vi "Periodic Tasks.vi"(8 "error in":errorcluster) -> ()   [LabVIEW 2018]
doc: "This VI runs in parallel to other tasks. It can contain as many user-defined periodic loops as you need. These can carry out PID or other sorts of timed response."
uses:
  SwerveRotationCalibrate.ctl
  <vilib>/Rock Robotics/WPI/ThirdParty/Phoenix-LabVIEW/Motor Controller/Controls/CTRE_Phoenix_MotorControl_NeutralMode.ctl
  <vilib>/Rock Robotics/WPI/ThirdParty/Phoenix-LabVIEW/Motor Controller/Controls/CTRE_Phoenix_MotorControl_ControlMode.ctl
  <vilib>/Rock Robotics/WPI/ThirdParty/Phoenix-LabVIEW/Motor Controller/Controls/CTRE_Phoenix_MotorControl_FeedbackDevice.ctl
  <vilib>/Rock Robotics/WPI/Utilities/WPI_GetSetVariantRefNum.vi
  <vilib>/Rock Robotics/Network Tables/NT Read Boolean.vi
  Robot Global Data.vi
  <vilib>/Rock Robotics/Network Tables/NT Write Numeric Array.vi
  d8969dce-e83f-414b-ab1b-b6caec8a5545.vi
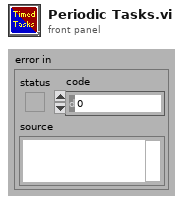
[diagram p1: front panel]
types:
  T1 = typedef "SwerveRotationCalibrate.ctl" = enum16{"Calibrate", "Home", "ResetQuad", "Drive"}
  T2 = typedef "CTRE_Phoenix_MotorControl_NeutralMode.ctl" = enum8{"EEPROMSetting", "Override to Coast", "Override to Brake"}
  T3 = typedef "CTRE_Phoenix_MotorControl_ControlMode.ctl" = u16
  T4 = typedef "CTRE_Phoenix_MotorControl_FeedbackDevice.ctl" = i8
  T5 = cluster{"T0":u32, "Mode":T1, "Rotation Neutral Mode":T2, "Rotation Control Mode":T3, "Feedback Device":T4}
  T6 = cluster{"Yaw":dbl, "Roll":dbl, "Pitch":dbl, "Heading":dbl, "Fused Heading":dbl}
  T7 = typedef "WPI_JoystickDevRef.ctl" = cluster{"Device":T8}
  T8 = typedef "WPI_JoystickDeviceEnum.ctl" = enum16{"USB 0", "USB 1", "USB 2", "USB 3", "USB 4", "USB 5"}
  T9 = typedef "WPI_DriverStationRobotMode2.ctl" = enum16{"Autonomous Disabled", "Autonomous Enabled", "Teleop Disabled", "Teleop Enabled", "Disconnected", "Finish", "Test Disabled", "Test Enabled", "Emergency Stopped"}
  T10 = cluster{"Buttons[0]":bool, "Buttons[1]":bool, "Buttons[2]":bool, "Buttons[3]":bool, "Buttons[4]":bool, "Buttons[5]":bool, "Buttons[6]":bool, "Buttons[7]":bool, "Buttons[8]":bool, "Buttons[9]":bool, "Buttons[10]":bool, "Buttons[11]":bool, "Buttons[12]":bool}
  T11 = cluster{"Motor1":cluster{"P":dbl, "I":dbl, "D":dbl}, "Motor3":cluster{"P":dbl, "I":dbl, "D":dbl}, "Motor2":cluster{"P":dbl, "I":dbl, "D":dbl}, "Motor4":cluster{"P":dbl, "I":dbl, "D":dbl}}
  T12 = typedef "WPI_CompressorDevRef.ctl" = cluster{"DevStatus":errorcluster, "Pneumatics Control Module":u8}
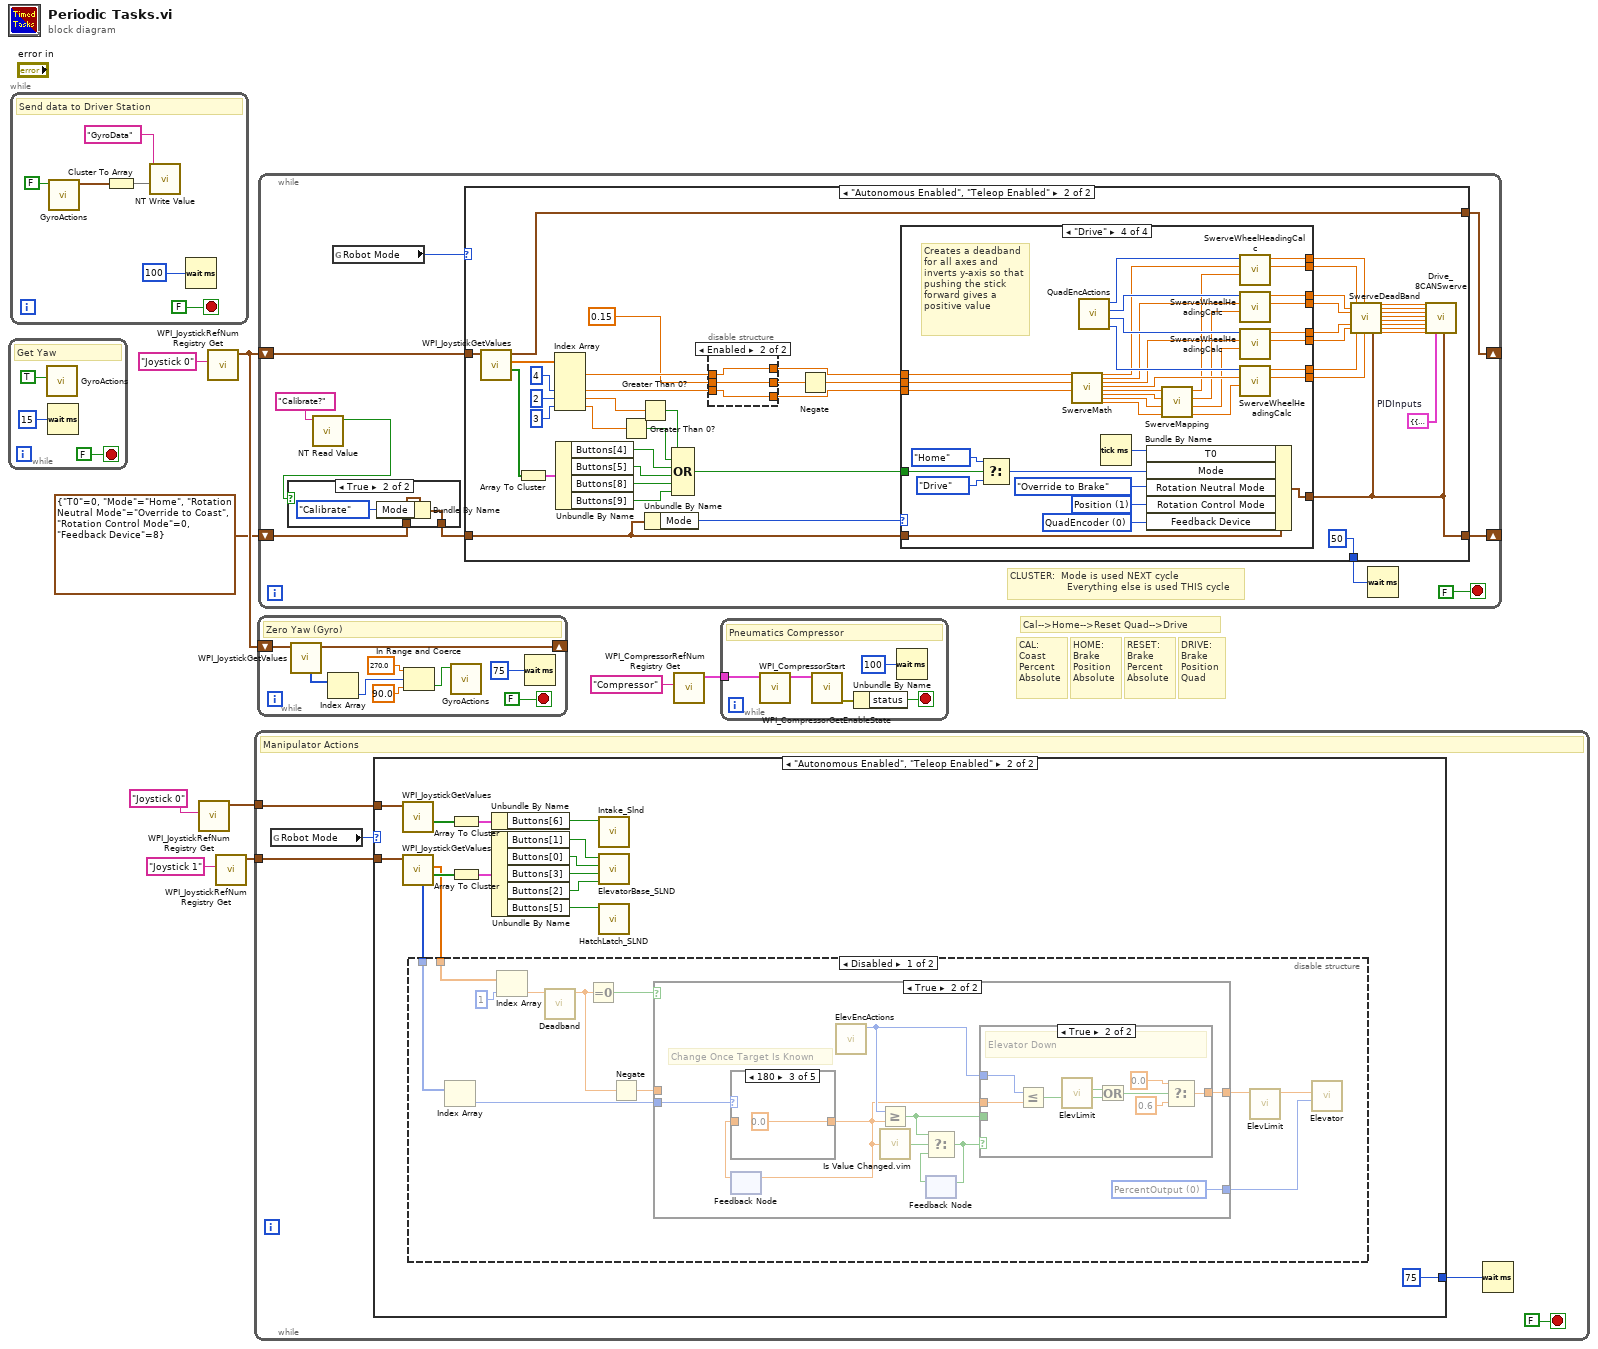
[diagram p0: block diagram]
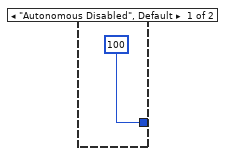
[diagram p2: hidden frame]
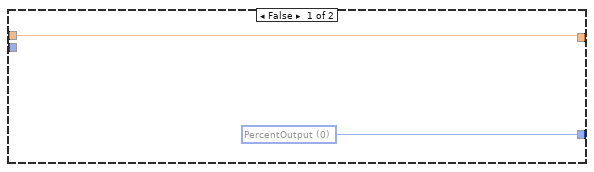
[diagram p3: hidden frame]
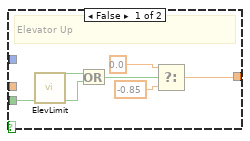
[diagram p4: hidden frame]
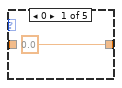
[diagram p5: hidden frame]
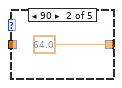
[diagram p6: hidden frame]
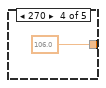
[diagram p7: hidden frame]
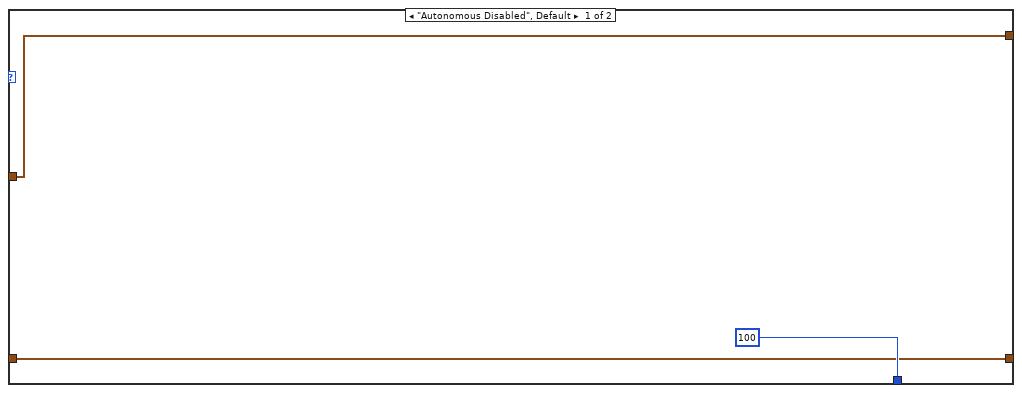
[diagram p11: hidden frame]
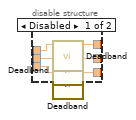
[diagram p12: hidden frame]
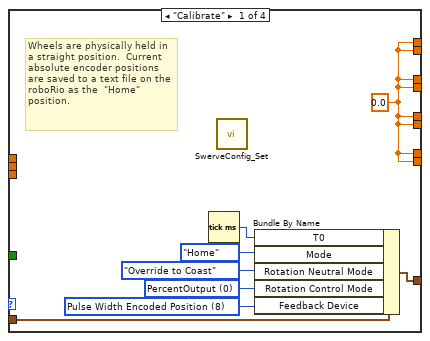
[diagram p13: hidden frame]
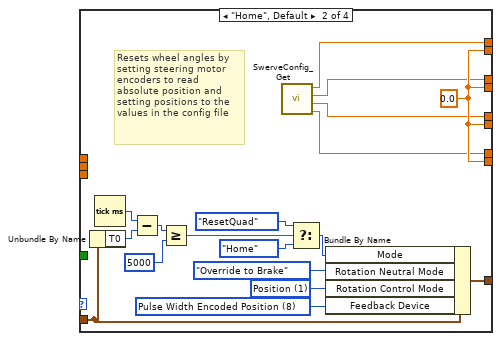
[diagram p14: hidden frame]
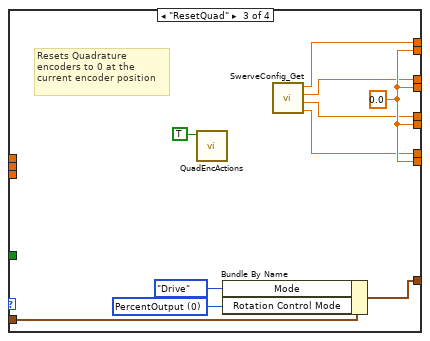
[diagram p15: hidden frame]
diagram:
  # "DRIVE:\nBrake\nPosition\nQuad"
  # "RESET:\nBrake\nPercent\nAbsolute"
  # "HOME:\nBrake\nPosition\nAbsolute"
  # "Cal-->Home-->Reset Quad-->Drive"
  # "CAL:\nCoast\nPercent\nAbsolute"
  n1 = while {
    stop <- FALSE stop-if-true
    # "Get Yaw"
    n2 = call "GyroActions.vi"("Update?"=TRUE ("Zero")) -> ()  [unwired: 9 in, 2 out]
    n3 = Wait (ms)(milliseconds to wait=u32 15) -> ()  [unwired: 1 out]
  }
  n4 = while {
    stop <- FALSE stop-if-true
    # "Send data to Driver Station"
    n5 = call "GyroActions.vi"("Zero"=FALSE) -> ("YRPHfH"=w16:T6)  [unwired: 9 in, 1 out]
    n6 = Cluster To Array(cluster=w16) -> (array=w15:dbl[])
    n7 = call-poly <vilib>:"NT Write Value.vi"("Numeric Array"=w15, "Name"="GyroData") -> ()  [unwired: 9 in, 1 out]
    n8 = Wait (ms)(milliseconds to wait=u32 100 ("millisecond timer value")) -> ()  [unwired: 1 out]
  }
  n9 = call <vilib>:"WPI_JoystickRefNum Registry Get.vi"("refnum name"="Joystick 0") -> ("JoystickDevRef"=w1:T7)  [unwired: 1 in, 9 out]
  n10 = call <vilib>:"WPI_JoystickRefNum Registry Get.vi"("refnum name"="Joystick 0") -> ("JoystickDevRef"=w8:T7)  [unwired: 1 in, 9 out]
  n11 = call <vilib>:"WPI_JoystickRefNum Registry Get.vi"("refnum name"="Joystick 1") -> ("JoystickDevRef"=w5:T7)  [unwired: 1 in, 9 out]
  n12 = while {
    tunnel: w5 -> [w22]
    tunnel: w1 -> [w19]
    stop <- FALSE stop-if-true
    # "Manipulator Actions"
    n13 = global read "Robot Global Data.vi" "Robot Mode"() -> (w23:T9)
    n14 = case shown="\"Autonomous Enabled\", \"Teleop Enabled\"" w23 {
      tunnel: w22 -> [_ w38]
      tunnel: [u32 100 ("milliseconds to wait") u32 75 ("milliseconds to wait")] -> w20
      tunnel: w19 -> [_ w26]
      frame "Autonomous Disabled", Default {
      }
      frame "Autonomous Enabled", "Teleop Enabled" {
        n15 = call <vilib>:"WPI_JoystickGetValues.vi"("JoystickDevRef"=w26) -> ("Buttons"=w27:bool[])  [unwired: 6 in, 4 out]
        n16 = call <vilib>:"WPI_JoystickGetValues.vi"("JoystickDevRef"=w38) -> ("Buttons"=w37:bool[], "Axes"=w30:dbl[], "POVs"=w29:i16[])  [unwired: 6 in, 2 out]
        n17 = disable-structure shown="Disabled" {
          disable-tunnel: w30 -> [w41 _]
          disable-tunnel: w29 -> [w40 _]
          frame Disabled {
            n18 = Index Array(array=w40) -> (element=w43:i16)  [unwired: 1 in]
            n19 = Index Array(array=w41, index=1) -> (element=w44:dbl)
            n20 = call "Deadband.vi"("Input"=w44) -> ("Output"=w50:dbl)  [unwired: 6 in]
            n21 = Equal To 0?(x=w50) -> (x = 0?=w45:bool)
            n22 = Negate(x=w50) -> (-x=w47:dbl)
            n23 = case shown="True" w45 {
              tunnel: w47 -> [w51 _]
              tunnel: w43 -> [_ w62]
              tunnel: [w52 w61] -> w46
              tunnel: [w51 w60] -> w48
              frame False {
                w52 = T3 0 items=["PercentOutput"=0, "Position"=1, "Velocity"=2, "Current"=3, "Follower"=5, "MotionProfile"=6, "MotionMagic"=7, "MotionProfileArc"=10, "Disabled"=15] ("Rotation Control Mode")
              }
              frame True {
                w61 = T3 0 items=["PercentOutput"=0, "Position"=1, "Velocity"=2, "Current"=3, "Follower"=5, "MotionProfile"=6, "MotionMagic"=7, "MotionProfileArc"=10, "Disabled"=15] ("Rotation Control Mode")
                # "Change Once Target Is Known"
                n24 = feedback #1() -> (w58:dbl)  [unwired: 1 in]
                n25 = case shown="180" w62 {
                  tunnel: [0.0 ("Target") 64.0 ("Target") 0.0 ("Target") 106.0 ("Target") w81] -> w57
                  tunnel: w58 -> [_ _ _ _ w81]
                  frame 0 {
                  }
                  frame 90 {
                  }
                  frame 180 {
                  }
                  frame 270 {
                  }
                  frame -1, Default {
                  }
                }
                n26 = feedback-in #1(w57) -> ()
                n27 = call "ElevEncActions.vi"() -> ("ElevEncPos"=w59:i32)  [unwired: 11 in]
                n28 = Greater Or Equal?(x=w59, y=w57) -> (x >= y?=w53:bool)
                n29 = call "Is Value Changed.vim"("value"=w57) -> ("changed or first call?"=w56:bool)
                n30 = feedback #2() -> (w55:bool)  [unwired: 1 in]
                n31 = Select(t=w53, s=w56, f=w55) -> (s? t:f=w54:bool)
                n32 = feedback-in #2(w54) -> ()
                n33 = case shown="True" w54 {
                  tunnel: [w65 w71] -> w60
                  tunnel: w57 -> [_ w73]
                  tunnel: w59 -> [_ w69]
                  tunnel: w53 -> [w63 _]
                  frame False {
                    # "Elevator Up"
                    n34 = call "ElevLimit.vi"() -> ("UpLimit"=w64:bool)  [unwired: 9 in, 2 out]
                    n35 = Or(x=w64, y=w63) -> (x .or. y?=w66:bool)
                    n36 = Select(t=0.0, s=w66, f=-0.85) -> (s? t:f=w65:dbl)
                  }
                  frame True {
                    # "Elevator Down"
                    n37 = Less Or Equal?(x=w69, y=w73) -> (x <= y?=w72:bool)
                    n38 = call "ElevLimit.vi"() -> ("BotLimit"=w70:bool)  [unwired: 9 in, 2 out]
                    n39 = Or(x=w70, y=w72) -> (x .or. y?=w74:bool)
                    n40 = Select(t=0.0, s=w74, f=0.6) -> (s? t:f=w71:dbl)
                  }
                }
              }
            }
            n41 = call "ElevLimit.vi"("PowerIn"=w48) -> ("PowerOut"=w49:dbl)  [unwired: 8 in, 2 out]
            n42 = call "Elevator.vi"("Control Mode"=w46, "Target"=w49) -> ()  [unwired: 10 in]
          }
          frame Enabled {
          }
        }
        n43 = Array To Cluster(array=w27) -> (cluster=w28:T10)
        n44 = Array To Cluster(array=w37) -> (cluster=w39:T10)
        n45 = Unbundle By Name(w28) -> ("Buttons[6]"=w25:bool)
        n46 = Unbundle By Name(w39) -> ("Buttons[1]"=w36:bool, "Buttons[0]"=w35:bool, "Buttons[3]"=w34:bool, "Buttons[2]"=w33:bool, "Buttons[5]"=w31:bool)
        n47 = call "Intake_Slnd.vi"("Toggle?"=w25) -> ()  [unwired: 11 in]
        n48 = call "ElevatorBase_SLND.vi"("CargoPick"=w33, "CargoDeliv"=w34, "Carry"=w35, "Hatch"=w36) -> ()  [unwired: 8 in]
        n49 = call "HatchLatch_SLND.vi"("Toggle?"=w31) -> ()  [unwired: 11 in]
      }
    }
    n50 = Wait (ms)(milliseconds to wait=w20) -> ()  [unwired: 1 out]
  }
  n51 = while {
    shift-right: [w83] -> _
    shift-left: w8 -> [w90]
    stop <- FALSE stop-if-true
    # "Zero Yaw (Gyro)"
    n52 = call <vilib>:"WPI_JoystickGetValues.vi"("JoystickDevRef"=w90) -> ("JoystickDevRef"=w83:T7, "POVs"=w88:i16[])  [unwired: 6 in, 3 out]
    n53 = Index Array(array=w88) -> (element=w87:i16)  [unwired: 1 in]
    n54 = In Range and Coerce(upper limit=270.0, x=w87, lower limit=90.0) -> (In Range?=w86:bool)  [unwired: 1 out]
    n55 = call "GyroActions.vi"("Zero"=w86) -> ()  [unwired: 9 in, 2 out]
    n56 = Wait (ms)(milliseconds to wait=u32 75) -> ()  [unwired: 1 out]
  }
  n57 = while {
    shift-right: [w98] -> _
    shift-left: w8 -> [w99]
    shift-right: [w97] -> _
    shift-left: T5 {"T0"=0, "Mode"=enum."Home", "Rotation Neutral Mode"=enum."Override to Coast", "Rotation Control Mode"=0, "Feedback Device"=8} ("RotationSettings") -> [w93]
    stop <- FALSE stop-if-true
    # "CLUSTER:  Mode is used NEXT cycle\n                   Everything else is used THIS cycle"
    n58 = call-poly <vilib>:"NT Read Value.vi"("Name"="Calibrate?") -> ("Boolean"=w91:bool)  [unwired: 9 in, 1 out]
    n59 = case shown="True" w91 {
      tunnel: w93 -> [w101 w104]
      tunnel: [w101 w103] -> w92
      frame False {
      }
      frame True {
        n60 = Bundle By Name(cluster=w104, "Mode"=SwerveRotationCalibrate."Calibrate") -> (w103:T5)
      }
    }
    n61 = global read "Robot Global Data.vi" "Robot Mode"() -> (w95:T9)
    n62 = case shown="\"Autonomous Enabled\", \"Teleop Enabled\"" w95 {
      tunnel: w99 -> [w105 w152]
      tunnel: [w105 w151] -> w98
      tunnel: [w106 w109] -> w97
      tunnel: w92 -> [w106 w133]
      tunnel: [u32 100 ("milliseconds to wait") u32 50 ("milliseconds to wait")] -> w96
      frame "Autonomous Disabled", Default {
      }
      frame "Autonomous Enabled", "Teleop Enabled" {
        w134 = T11 {"Motor1"={"P"=4.0, "I"=0.0, "D"=64.0}, "Motor3"={"P"=4.0, "I"=0.0, "D"=64.0}, "Motor2"={"P"=4.0, "I"=0.0, "D"=64.0}, "Motor4"={"P"=4.0, "I"=0.0, "D"=64.0}}  # PIDInputs
        n63 = call <vilib>:"WPI_JoystickGetValues.vi"("JoystickDevRef"=w152) -> ("Buttons"=w148:bool[], "Axes"=w150:dbl[], "JoystickDevRef"=w151:T7)  [unwired: 6 in, 2 out]
        n64 = Array To Cluster(array=w148) -> (cluster=w147:T10)
        n65 = Index Array(array=w150, index #3=4 ("index"), index #4=2 ("index"), index #5=3 ("index")) -> (element #1=w135:dbl, element #3=w136:dbl, element #4=w141:dbl, element #5=w142:dbl)  [unwired: 2 in, 1 out]
        n66 = Unbundle By Name(w147) -> ("Buttons[4]"=w137:bool, "Buttons[5]"=w138:bool, "Buttons[8]"=w140:bool, "Buttons[9]"=w139:bool)
        n67 = Greater Than 0?(x=w142) -> (x > 0?=w144:bool)
        n68 = Greater Than 0?(x=w141) -> (x > 0?=w143:bool)
        n69 = Unbundle By Name(w133) -> ("Mode"=w132:T1)
        n70 = Compound Arithmetic op=OR(w143, w144, w137, w138, w140, w139) -> (w131:bool)
        n71 = disable-structure shown="Enabled" {
          disable-tunnel: w136 -> [w158 w159]
          disable-tunnel: 0.15 ("upper limit") -> [w157 w160]
          disable-tunnel: w135 -> [w156 w161]
          disable-tunnel: [w155 w160] -> w129
          disable-tunnel: [w154 w159] -> w127
          disable-tunnel: [w153 w161] -> w126
          frame Disabled {
            n72 = call "Deadband.vi"("Input"=w156) -> ("Output"=w153:dbl)  [unwired: 6 in]
            n73 = call "Deadband.vi"("Input"=w157) -> ("Output"=w155:dbl)  [unwired: 6 in]
            n74 = call "Deadband.vi"("Input"=w158) -> ("Output"=w154:dbl)  [unwired: 6 in]
          }
          frame Enabled {
          }
        }
        n75 = Negate(x=w129) -> (-x=w128:dbl)
        n76 = case shown="\"Drive\"" w132 {
          tunnel: [w163 w187 w193 w230] -> w122
          tunnel: [w163 w186 w188 w224] -> w125
          tunnel: [w163 w187 w193 w228] -> w124
          tunnel: [w163 w185 w189 w229] -> w123
          tunnel: [w163 w187 w193 w234] -> w118
          tunnel: [w163 w184 w191 w233] -> w119
          tunnel: [w163 w187 w193 w232] -> w121
          tunnel: [w163 w183 w190 w231] -> w120
          tunnel: w133 -> [w169 w175 w197 w210]
          tunnel: [w167 w179 w196 w208] -> w109
          tunnel: w131 -> [_ _ _ w205]
          tunnel: w128 -> [_ _ _ w200]
          tunnel: w127 -> [_ _ _ w199]
          tunnel: w126 -> [_ _ _ w198]
          frame "Calibrate" {
            w163 = 0.0 ("P")
            w166 = T3 0 items=["PercentOutput"=0, "Position"=1, "Velocity"=2, "Current"=3, "Follower"=5, "MotionProfile"=6, "MotionMagic"=7, "MotionProfileArc"=10, "Disabled"=15] ("Rotation Control Mode")
            w168 = T4 8 items=["None"=-1, "QuadEncoder"=0, "Analog"=2, "Tachometer"=4, "Pulse Width Encoded Position"=8, "Sensor Sum (S0 + S1)"=9, "Sensor Difference (D0 - D1)"=10, "Remote Source 0"=11, "Remote Source 1"=12, "Software Emulated"=15] ("Feedback Device")
            # "Wheels are physically held in a straight position.  Current absolute encoder positions are saved to a text file on the roboRio as the  \"Home\" position."
            n77 = Tick Count (ms)() -> (millisecond timer value=w162:u32)
            n78 = call "SwerveConfig_Set.vi"() -> ()  [unwired: 12 in]
            n79 = Bundle By Name(cluster=w169, "T0"=w162, "Mode"=SwerveRotationCalibrate."Home", "Rotation Neutral Mode"=CTRE_Phoenix_MotorControl_NeutralMode."Override to Coast", "Rotation Control Mode"=w166, "Feedback Device"=w168) -> (w167:T5)
          }
          frame "Home", Default {
            w181 = T3 1 items=["PercentOutput"=0, "Position"=1, "Velocity"=2, "Current"=3, "Follower"=5, "MotionProfile"=6, "MotionMagic"=7, "MotionProfileArc"=10, "Disabled"=15] ("Rotation Control Mode")
            w182 = T4 8 items=["None"=-1, "QuadEncoder"=0, "Analog"=2, "Tachometer"=4, "Pulse Width Encoded Position"=8, "Sensor Sum (S0 + S1)"=9, "Sensor Difference (D0 - D1)"=10, "Remote Source 0"=11, "Remote Source 1"=12, "Software Emulated"=15] ("Feedback Device")
            w187 = 0.0 ("P")
            # "Resets wheel angles by setting steering motor encoders to read absolute position and setting positions to the values in the config file"
            n80 = Unbundle By Name(w175) -> ("T0"=w173:u32)
            n81 = Tick Count (ms)() -> (millisecond timer value=w174:u32)
            n82 = Subtract(x=w174, y=w173) -> (x-y=w172:u32)
            n83 = Greater Or Equal?(x=w172, y=u32 5000) -> (x >= y?=w171:bool)
            n84 = call "SwerveConfig_Get.vi"() -> ("RearRightHome"=w184:dbl, "RearLeftHome"=w183:dbl, "FrontRightHome"=w185:dbl, "FrontLeftHome"=w186:dbl)  [unwired: 8 in]
            n85 = Select(t=SwerveRotationCalibrate."ResetQuad" ("Mode"), s=w171, f=SwerveRotationCalibrate."Home" ("Mode")) -> (s? t:f=w178:T1)
            n86 = Bundle By Name(cluster=w175, "Mode"=w178, "Rotation Neutral Mode"=CTRE_Phoenix_MotorControl_NeutralMode."Override to Brake", "Rotation Control Mode"=w181, "Feedback Device"=w182) -> (w179:T5)
          }
          frame "ResetQuad" {
            w194 = T3 0 items=["PercentOutput"=0, "Position"=1, "Velocity"=2, "Current"=3, "Follower"=5, "MotionProfile"=6, "MotionMagic"=7, "MotionProfileArc"=10, "Disabled"=15] ("Rotation Control Mode")
            w193 = 0.0 ("P")
            # "Resets Quadrature encoders to 0 at the current encoder position"
            n87 = call "QuadEncActions.vi"("Zero?"=TRUE ("Reset?")) -> ()  [unwired: 7 in, 4 out]
            n88 = Bundle By Name(cluster=w197, "Mode"=SwerveRotationCalibrate."Drive", "Rotation Control Mode"=w194) -> (w196:T5)
            n89 = call "SwerveConfig_Get.vi"() -> ("RearRightHome"=w191:dbl, "RearLeftHome"=w190:dbl, "FrontRightHome"=w189:dbl, "FrontLeftHome"=w188:dbl)  [unwired: 8 in]
          }
          frame "Drive" {
            w207 = T3 1 items=["PercentOutput"=0, "Position"=1, "Velocity"=2, "Current"=3, "Follower"=5, "MotionProfile"=6, "MotionMagic"=7, "MotionProfileArc"=10, "Disabled"=15] ("Rotation Control Mode")
            w209 = T4 0 items=["None"=-1, "QuadEncoder"=0, "Analog"=2, "Tachometer"=4, "Pulse Width Encoded Position"=8, "Sensor Sum (S0 + S1)"=9, "Sensor Difference (D0 - D1)"=10, "Remote Source 0"=11, "Remote Source 1"=12, "Software Emulated"=15] ("Feedback Device")
            # "Creates a deadband for all axes and inverts y-axis so that pushing the stick forward gives a positive value"
            n90 = Select(t=SwerveRotationCalibrate."Home" ("Mode"), s=w205, f=SwerveRotationCalibrate."Drive" ("Mode")) -> (s? t:f=w202:T1)
            n91 = call "SwerveMath.vi"("X-Axis"=w198, "Y-Axis"=w200, "Turn"=w199) -> ("FrontLeftAngle"=w219:dbl, "FrontRightAngle"=w220:dbl, "RearLeftAngle"=w221:dbl, "RearRightAngle"=w222:dbl, "FrontLeftDrive"=w218:dbl, "FrontRightDrive"=w217:dbl, "RearLeftDrive"=w216:dbl, "RearRightDrive"=w215:dbl)  [unwired: 17 in]
            n92 = call "QuadEncActions.vi"() -> ("RearRightQuadPos"=w226:i32, "RearLeftQuadPos"=w225:i32, "FrontRightQuadPos"=w227:i32, "FrontLeftQuadPos"=w223:i32)  [unwired: 8 in]
            n93 = Tick Count (ms)() -> (millisecond timer value=w201:u32)
            n94 = Bundle By Name(cluster=w210, "T0"=w201, "Mode"=w202, "Rotation Neutral Mode"=CTRE_Phoenix_MotorControl_NeutralMode."Override to Brake", "Rotation Control Mode"=w207, "Feedback Device"=w209) -> (w208:T5)
            n95 = call "SwerveMapping.vi"("RearRightDriveIn"=w215, "RearLeftDriveIn"=w216, "FrontRightDriveIn"=w217, "FrontLeftDriveIn"=w218) -> ("RearRightDriveOut"=w211:dbl, "RearLeftDriveOut"=w212:dbl, "FrontRightDriveOut"=w213:dbl, "FrontLeftDriveOut"=w214:dbl)  [unwired: 4 in]
            n96 = call "SwerveWheelHeadingCalc.vi"("DriveIn"=w214, "Target"=w219, "Current"=w223) -> ("DriveOut"=w228:dbl, "TargetFinal"=w224:dbl)  [unwired: 7 in]
            n97 = call "SwerveWheelHeadingCalc.vi"("DriveIn"=w213, "Target"=w220, "Current"=w227) -> ("DriveOut"=w230:dbl, "TargetFinal"=w229:dbl)  [unwired: 7 in]
            n98 = call "SwerveWheelHeadingCalc.vi"("DriveIn"=w212, "Target"=w221, "Current"=w225) -> ("DriveOut"=w232:dbl, "TargetFinal"=w231:dbl)  [unwired: 7 in]
            n99 = call "SwerveWheelHeadingCalc.vi"("DriveIn"=w211, "Target"=w222, "Current"=w226) -> ("DriveOut"=w234:dbl, "TargetFinal"=w233:dbl)  [unwired: 7 in]
          }
        }
        n100 = call "SwerveDeadBand.vi"("FrontRightRotationIn"=w123, "FrontRightDriveIn"=w122, "RearLeftRotationIn"=w120, "RearLeftDriveIn"=w121, "FrontLeftDriveIn"=w124, "RearRightRotationIn"=w119, "FrontLeftRotationIn"=w125, "RearRightDriveIn"=w118, "RotationSettings"=w109) -> ("FrontLeftRotationOut"=w117:dbl, "FrontLeftDriveOut"=w116:dbl, "FrontRightRotationOut"=w115:dbl, "FrontRightDriveOut"=w114:dbl, "RearLeftRotationOut"=w113:dbl, "RearLeftDriveOut"=w112:dbl, "RearRightRotationOut"=w111:dbl, "RearRightDriveOut"=w110:dbl)  [unwired: 11 in]
        n101 = call "Drive_8CANSwerve.vi"("FrontLeftRotation"=w117, "FrontLeftDrive"=w116, "FrontRightRotation"=w115, "FrontRightDrive"=w114, "RearLeftRotation"=w113, "RearLeftDrive"=w112, "RearRightRotation"=w111, "RearRightDrive"=w110, "PIDInputs"=w134, "RotationSettings"=w109) -> ()  [unwired: 18 in]
      }
    }
    n102 = Wait (ms)(milliseconds to wait=w96) -> ()  [unwired: 1 out]
  }
  n103 = call <vilib>:"WPI_CompressorRefNum Registry Get.vi"("refnum name"="Compressor") -> ("CompressorDevRef"=w3:T12)  [unwired: 9 in, 1 out]
  n104 = while {
    tunnel: w3 -> [w237]
    stop <- w238 stop-if-true
    # "Pneumatics Compressor"
    n105 = call <vilib>:"WPI_CompressorStart.vi"("CompressorDevRef"=w237) -> ("CompressorDevRef"=w236:T12)  [unwired: 9 in, 1 out]
    n106 = call <vilib>:"WPI_CompressorGetEnableState.vi"("CompressorDevRef"=w236) -> ("error out"=w235:errorcluster)  [unwired: 1 in, 9 out]
    n107 = Unbundle By Name(w235) -> ("status"=w238:bool)
    n108 = Wait (ms)(milliseconds to wait=u32 100) -> ()  [unwired: 1 out]
  }
